vi "Get File Data From Internet.vi"(5 "Error In":errorcluster, 6 "ms timeout (10000)":i32, 7 "URL to File":string) -> (1 "error out":errorcluster, 3 "File data":string)   [LabVIEW 2015]
uses:
  <vilib>/Utility/error.llb/Error Cluster From Error Code.vi
  <vilib>/ErrorRing/Error Ring.xnode
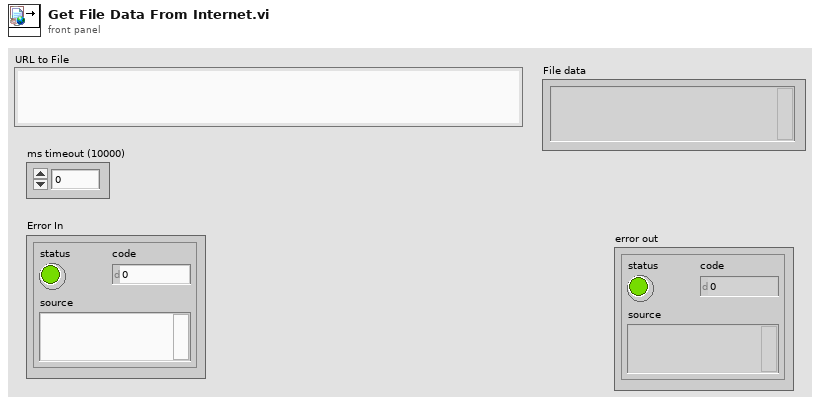
[diagram p1: front panel]
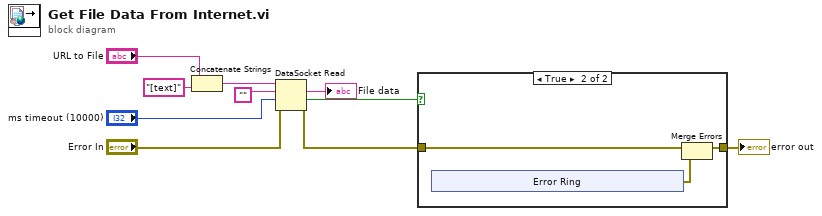
[diagram p0: block diagram]
diagram:
  n1 = Concatenate Strings("URL to File", "[text]" ("string")) -> (w9:string)
  n2 = DataSocket Read(8:"Error In", 9:"ms timeout (10000)", 10:"", 11:w9) -> (0:w2:errorcluster, 1:w3:bool, 2:→"File data":string)  [unwired: 1 in, 4 out]
  n3 = case shown="True" w3 {
    tunnel: w2 -> [w11 w14]
    tunnel: [w11 w12] -> w1
    frame False {
    }
    frame True {
      n4 = xnode "Error Ring"() -> ("error out"=w13:errorcluster)
      n5 = Merge Errors(w14, w13) -> (w12:errorcluster)
    }
  }
  "error out" <- w1
